vi "Phasor Convert (g,s,f) to (tf, tm).vi"(6 "IRF offset (t0)":dbl[unit] format="%#.3e", 8 "Error In":errorcluster, 9 "Phasor Harmonic Frequency":dbl[unit], 10 "Phasor (g, s)":T1, 11 "z":cdb=nan+0.0i) -> (0 "Error Out":errorcluster, 1 "Modulus Lifetime":dbl[unit] format="%#.3e", 2 "Phase Lifetime":dbl[unit] format="%#.3e")   [LabVIEW 2021, in "Phasor.lvlib"]
uses:
  Phasor.lvlib
  Phasor (g, s).ctl
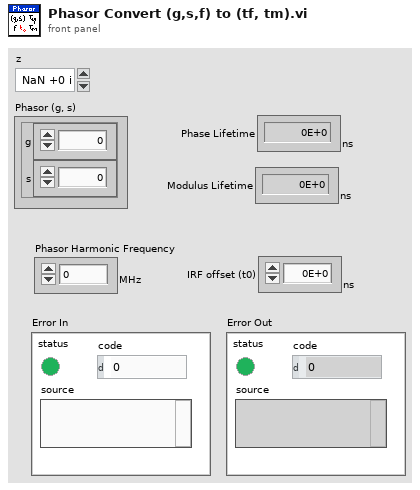
[diagram p1: front panel]
types:
  T1 = typedef "Phasor.lvlib/Phasor (g, s).ctl" = cluster{"g":dbl, "s":dbl}
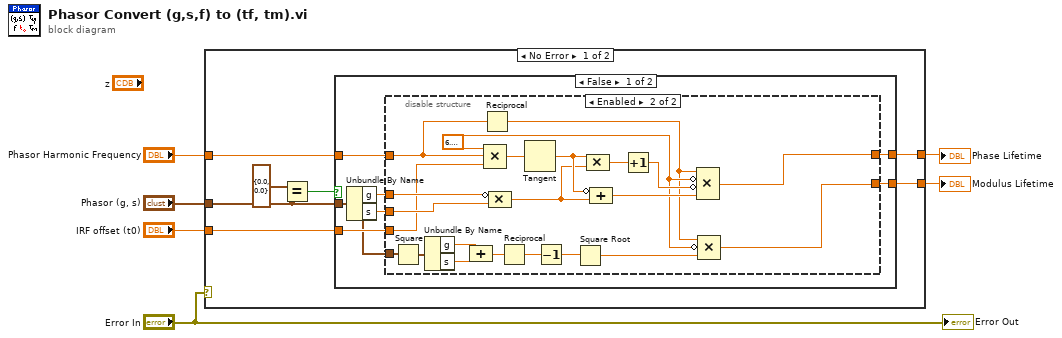
[diagram p0: block diagram]
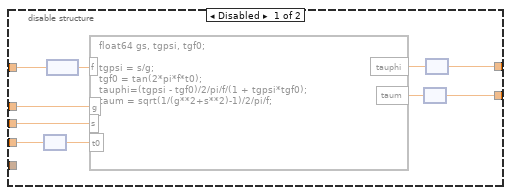
[diagram p2: hidden frame]
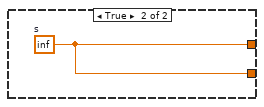
[diagram p3: hidden frame]
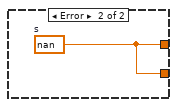
[diagram p4: hidden frame]
diagram:
  n1 = case shown="No Error" "Error In" {
    tunnel: "Phasor Harmonic Frequency" -> [w13 _]
    tunnel: [w12 w54] -> w5
    tunnel: [w11 w54] -> w4
    tunnel: "IRF offset (t0)" -> [w10 _]
    tunnel: "Phasor (g, s)" -> [w9 _]
    frame No Error {
      n2 = Equal?(x=T1 {"g"=0.0, "s"=0.0}, y=w9) -> (x = y?=w7:bool)
      n3 = case shown="False" w7 {
        tunnel: w13 -> [w18 _]
        tunnel: [w17 w53] -> w12
        tunnel: [w16 w53] -> w11
        tunnel: w10 -> [w15 _]
        tunnel: w9 -> [w14 _]
        frame False {
          n4 = Unbundle By Name(w14) -> ("g"=w19:dbl, "s"=w20:dbl)
          n5 = disable-structure shown="Enabled" {
            disable-tunnel: w20 -> [w30 w51]
            disable-tunnel: w19 -> [w29 w52]
            disable-tunnel: w18 -> [w26 w44]
            disable-tunnel: [w24 w42] -> w17
            disable-tunnel: [w23 w31] -> w16
            disable-tunnel: w15 -> [w22 w50]
            disable-tunnel: w14 -> [_ w41]
            frame Disabled {
              n6 = node(w22) -> (w21:dbl)
              n7 = node(w26) -> (w25:dbl)
              n8 = formula code="float64 gs, tgpsi, tgf0;\n\ntgpsi = s/g;\ntgf0 = tan(2*pi*f*t0);\ntauphi=(tgpsi - tgf0)/2/pi/f/(1 + tgpsi*tgf0);\ntaum = sqrt(1/(g**2+s**2)-1)/2/pi/f;"("f"=w25, "g"=w29, "s"=w30, "t0"=w21) -> ("tauphi"=w27:dbl, "taum"=w28:dbl)
              n9 = node(w28) -> (w23:dbl[unit])
              n10 = node(w27) -> (w24:dbl[unit])
            }
            frame Enabled {
              w33 = 6.283185307179586
              n11 = Square(x=w41) -> (x^2=w40:T1)
              n12 = Unbundle By Name(w40) -> ("g"=w39:dbl, "s"=w38:dbl)
              n13 = Compound Arithmetic op=ADD(w39, w38) -> (w37:dbl)
              n14 = Reciprocal(x=w44) -> (1/x=w32:dbl[unit])
              n15 = Compound Arithmetic op=MULTIPLY(w33, w44, w50) -> (w49:dbl)
              n16 = Compound Arithmetic op=MULTIPLY(invert w52, w51) -> (w47:dbl)
              n17 = Reciprocal(x=w37) -> (1/x=w36:dbl)
              n18 = Tangent(1:w49) -> (0:w48:dbl)
              n19 = Decrement(x=w36) -> (x-1=w35:dbl)
              n20 = Square Root(x=w35) -> (sqrt(x)=w34:dbl)
              n21 = Compound Arithmetic op=MULTIPLY(w48, w47) -> (w46:dbl)
              n22 = Compound Arithmetic op=ADD(invert w48, w47) -> (w45:dbl)
              n23 = Increment(x=w46) -> (x+1=w43:dbl)
              n24 = Compound Arithmetic op=MULTIPLY(w32, invert w33, invert w43, w45) -> (w42:dbl[unit])
              n25 = Compound Arithmetic op=MULTIPLY(w32, invert w33, w34) -> (w31:dbl[unit])
            }
          }
        }
        frame True {
          w53 = dbl[unit] inf  # s
        }
      }
    }
    frame Error {
      w54 = dbl[unit] nan  # s
    }
  }
  "Phase Lifetime" <- w5
  "Modulus Lifetime" <- w4
  "Error Out" <- "Error In"
